vi "Import Invoice data.vi"(0 "Refnum in":T2, 1 "iqa":string, 2 "item_data":T3, 3 "item_data_name":string[](array[string]), 4 "Invoive date":string, 5 "Item no":string, 6 "File data in":string[][](array[string]), 7 "Import Data":T1, 8 "row data":string[](array[string]), 10 "index":i32, 12 "item":string) -> (14 "Refnum out":T2, 15 "File data out":string[][](array[string]), 19 "error out":errorcluster)   [LabVIEW 2017]
uses:
  Control/item colum type.ctl
  <vilib>/addons/database/Connection.llb/Conn ObjectReference.ctl
  <vilib>/addons/database/Connection.llb/Conn Execute.vi
  <vilib>/addons/database/Recordset.llb/Rec Destroy - Connection.vi
  <vilib>/addons/database/Recordset.llb/Rec Fetch Recordset Data (R).vi
  <vilib>/addons/database/_DB Variant To Data/Database Variant To Data.xnode
  <vilib>/addons/database/NI_Database_API.lvlib
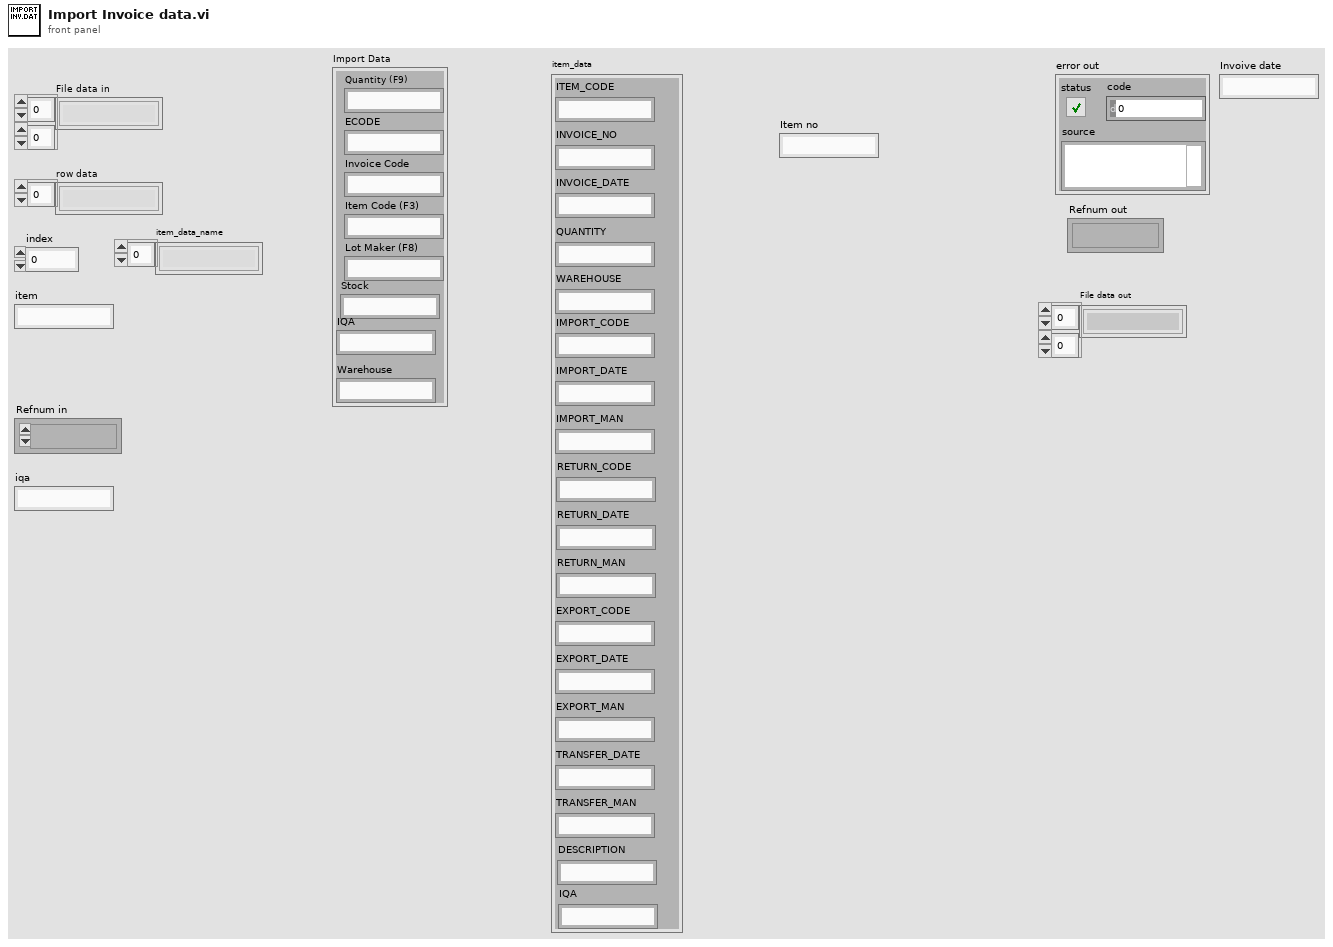
[diagram p1: front panel]
types:
  T1 = cluster{"Quantity (F9)":string, "ECODE":string, "Invoice Code":string, "Item Code (F3)":string, "Lot Maker (F8)":string, "Stock":string, "IQA":string, "Warehouse":string}
  T2 = typedef "NI_Database_API.lvlib/Conn ObjectReference.ctl" = refnum<k1>
  T3 = typedef "item colum type.ctl" = cluster{"ITEM_CODE":string, "INVOICE_NO":string, "INVOICE_DATE":string, "QUANTITY":string, "IMPORT_CODE":string, "IMPORT_DATE":string, "IMPORT_MAN":string, "RETURN_CODE":string, "RETURN_DATE":string, "RETURN_MAN":string, "EXPORT_CODE":string, "EXPORT_DATE":string, "EXPORT_MAN":string, "TRANSFER_DATE":string, "TRANSFER_MAN":string, "DESCRIPTION":string, "IQA":string, "WAREHOUSE":string}
  T4 = cluster{"Item Code (F3)":string, "Invoice Code":string, "Invoive date":string, "Quantity (F9)":string, "Item no":string, "IQA":string, "Lot Maker (F8)":string, "Warehouse":string}
  T5 = typedef "NI_Database_API.lvlib/Rec ObjectReference.ctl" = refnum<k1>
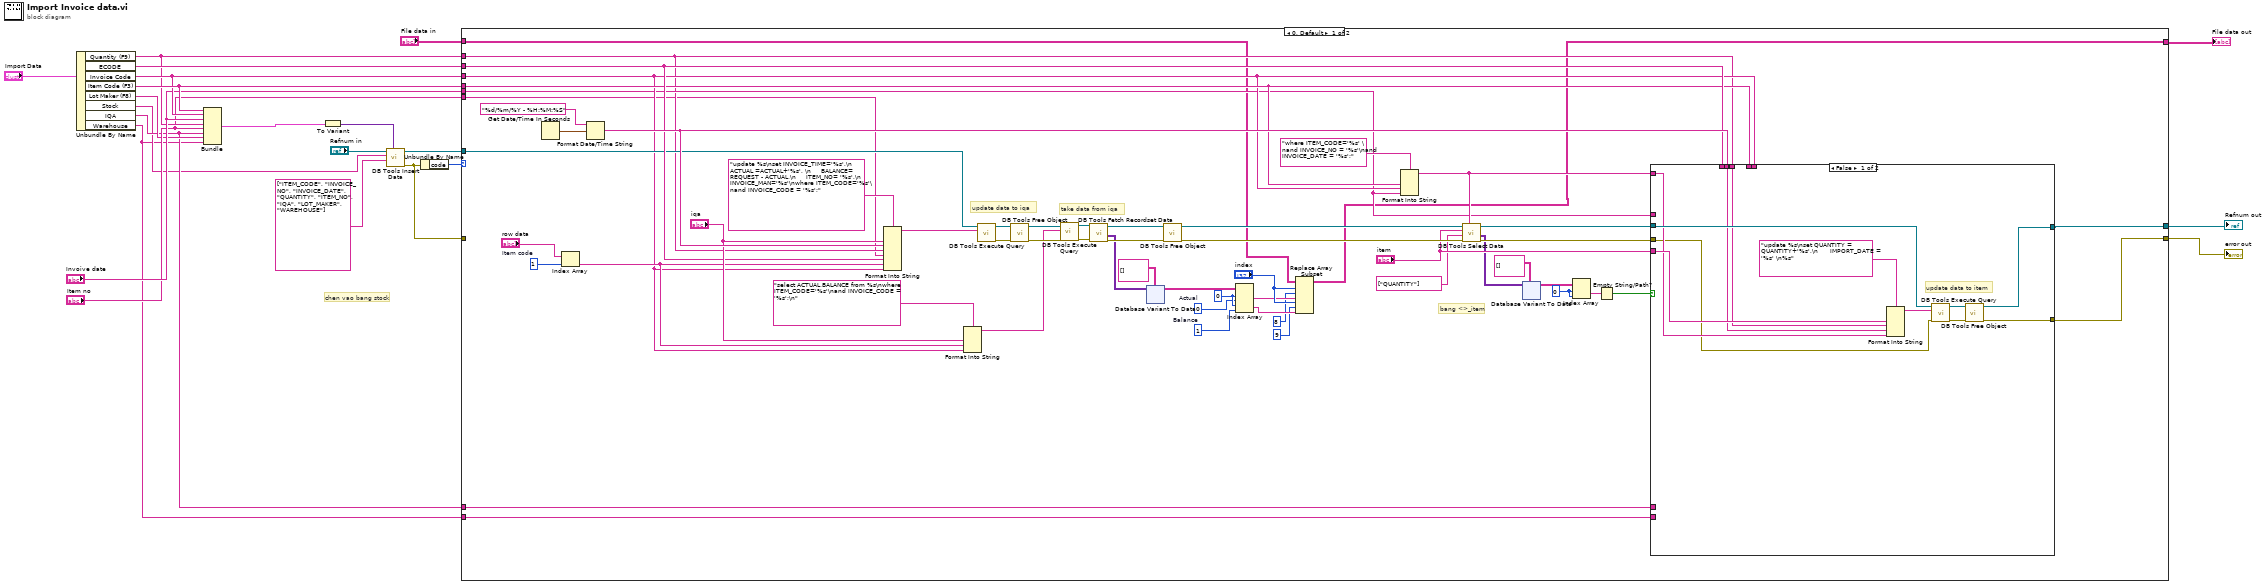
[diagram p0: block diagram]
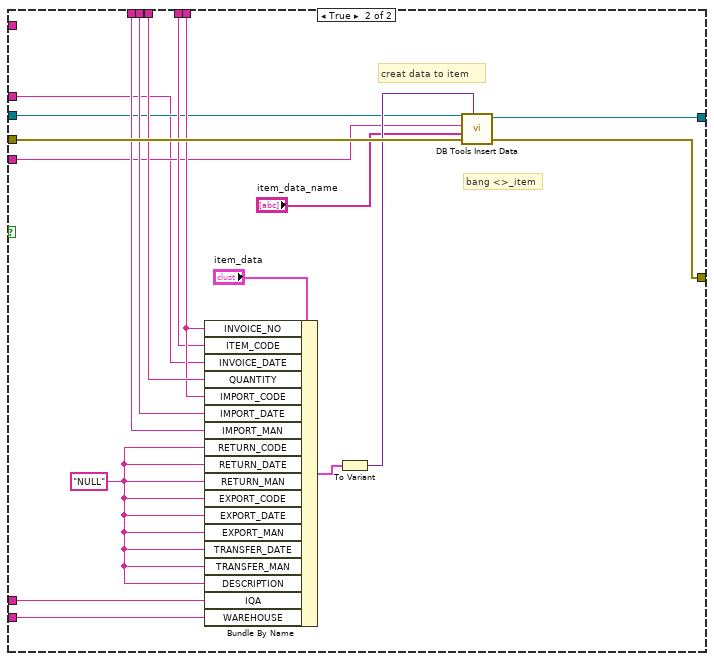
[diagram p2: hidden frame]
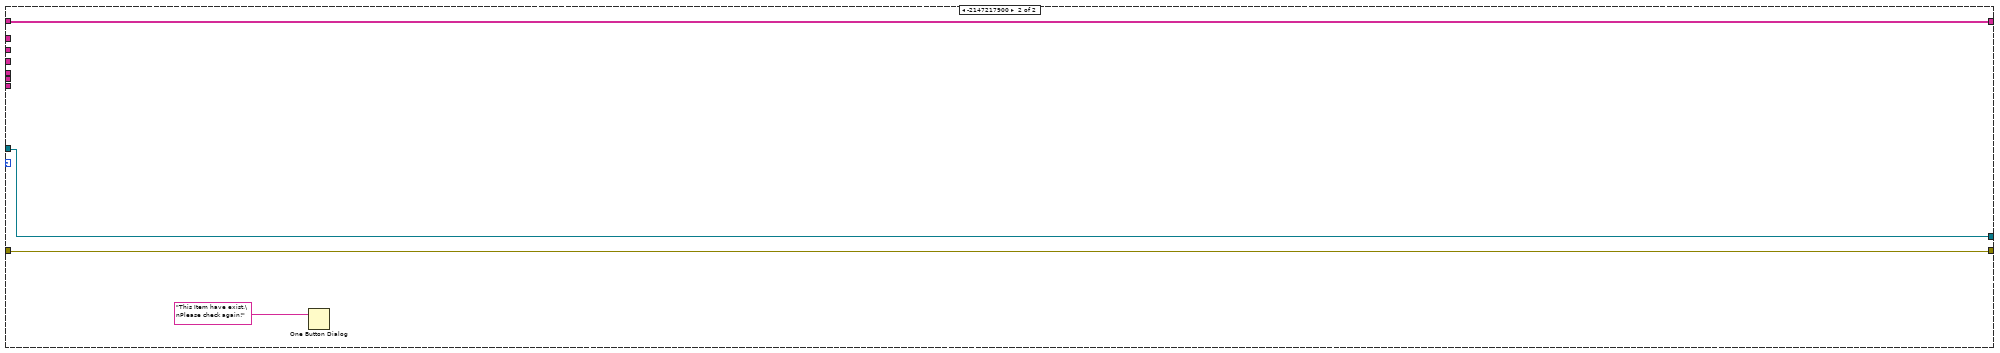
[diagram p3: hidden frame]
diagram:
  # "chen vao bang stock"
  n1 = Unbundle By Name("Import Data") -> ("Quantity (F9)"=w14:string, "ECODE"=w21:string, "Invoice Code"=w16:string, "Item Code (F3)"=w17:string, "Lot Maker (F8)"=w4:string, "Stock"=w2:string, "IQA"=w3:string, "Warehouse"=w1:string)
  n2 = Bundle("Item Code (F3)"=w17, "Invoice Code"=w16, "Invoive date"="Invoive date", "Quantity (F9)"=w14, "Item no"="Item no", "IQA"=w3, "Lot Maker (F8)"=w4, "Warehouse"=w1) -> (w13:T4)  [unwired: 1 in]
  n3 = To Variant(anything=w13) -> (Variant=w12:variant)
  n4 = call <vilib>:"DB Tools Insert Data.vi"("data"=w12, "columns"=string[] ["ITEM_CODE", "INVOICE_NO", "INVOICE_DATE", "QUANTITY", "ITEM_NO", "IQA", "LOT_MAKER", "WAREHOUSE"], "table"=w2, "connection reference"="Refnum in") -> ("error out"=w7:errorcluster, "connection reference out"=w19:T2)  [unwired: 6 in]
  n5 = Unbundle By Name(w7) -> ("code"=w11:i32)
  n6 = case shown="0, Default" w11 {
    tunnel: w21 -> [w46 _]
    tunnel: w19 -> [w34 w198]
    tunnel: w17 -> [w33 _]
    tunnel: w16 -> [w32 _]
    tunnel: "Invoive date" -> [w31 _]
    tunnel: w14 -> [w30 _]
    tunnel: "Item no" -> [w29 _]
    tunnel: w3 -> [w28 _]
    tunnel: "File data in" -> [w27 w199]
    tunnel: [w26 w198] -> w9
    tunnel: [w25 w199] -> w8
    tunnel: w7 -> [_ w197]
    tunnel: [w24 w197] -> w6
    tunnel: w1 -> [w23 _]
    frame 0, Default {
      w39 = 0 ("index (row)")
      w56 = 1  # Balance
      w55 = 0  # Actual
      w78 = 0 ("index (row)")
      w50 = 1  # Item code
      # "bang <>_item"
      # "take data from iqa"
      # "update data to iqa"
      n7 = Get Date/Time In Seconds() -> (seconds since 1Jan1904=w68:timestamp)
      n8 = Index Array(array="row data", index=w50) -> (element=w66:string)
      n9 = Format Date/Time String(time format string (%c)="%d/%m/%Y - %H:%M:%S", seconds (now)=w68) -> (date/time string=w72:string)  [unwired: 1 in]
      n10 = Format Into String(format string="update %s\nset INVOICE_TIME='%s',\n     ACTUAL =ACTUAL+'%s', \n     BALANCE= REQUEST - ACTUAL,\n     ITEM_NO= '%s',\n     INVOICE_MAN='%s'\nwhere ITEM_CODE='%s'\nand INVOICE_CODE = '%s';", "iqa", w72, w30, w29, w46, w66, w32) -> (resulting string=w64:string)  [unwired: 2 in, 1 out]
      n11 = Format Into String(format string="select ACTUAL,BALANCE from %s\nwhere ITEM_CODE='%s'\nand INVOICE_CODE = '%s';\n", "iqa", w66, w32) -> (resulting string=w67:string)  [unwired: 2 in, 1 out]
      n12 = call-poly <vilib>:"DB Tools Execute Query.vi"("SQL query"=w64, "connection reference"=w34) -> ("error out"=w73:errorcluster, "recordset reference"=w62:T5)  [unwired: 6 in]
      n13 = call-poly <vilib>:"DB Tools Free Object.vi"("error in (no error)"=w73, "recordset reference"=w62) -> ("error out"=w74:errorcluster, "connection reference"=w63:T2)  [unwired: 8 in]
      n14 = call-poly <vilib>:"DB Tools Execute Query.vi"("error in (no error)"=w74, "SQL query"=w67, "connection reference"=w63) -> ("error out"=w75:errorcluster, "recordset reference"=w47:T5)  [unwired: 5 in]
      n15 = call-poly <vilib>:"DB Tools Fetch Recordset Data.vi"("error in (no error)"=w75, "recordset reference"=w47) -> ("error out"=w76:errorcluster, "recordset data"=w51:variant[][], "recordset reference out"=w48:T5)  [unwired: 3 in]
      n16 = xnode "Database Variant To Data"("database variant"=w51, "type"=string[][] []) -> ("data"=w53:string[][])  [unwired: 1 in, 1 out]
      n17 = call-poly <vilib>:"DB Tools Free Object.vi"("error in (no error)"=w76, "recordset reference"=w48) -> ("error out"=w77:errorcluster, "connection reference"=w71:T2)  [unwired: 8 in]
      n18 = Index Array(array=w53, index (row) #1=w78, index (col) #1=w55, index (row) #2=w78, index (col) #2=w56) -> (element #1=w59:string, element #2=w60:string)
      n19 = Replace Array Subset "Replace Array Subset"(array=w27, new element #1=w59, index (row) #1="index", index (col) #1=8 ("disabled index (col)"), new element #2=w60, index (row) #2="index", index (col) #2=9 ("disabled index (col)")) -> (w25:string[][])
      n20 = Format Into String(format string="where ITEM_CODE='%s' \nand INVOICE_NO = '%s'\nand INVOICE_DATE = '%s';" ("condition"), w33, w32, w31) -> (resulting string=w35:string)  [unwired: 2 in, 1 out]
      n21 = call <vilib>:"DB Tools Select Data.vi"("condition"=w35, "columns"=string[] ["QUANTITY"], "table"="item", "connection reference"=w71) -> ("data"=w41:variant[][], "connection reference out"=w45:T2)  [unwired: 2 in, 1 out]
      n22 = xnode "Database Variant To Data"("database variant"=w41, "type"=string[][] []) -> ("data"=w40:string[][])  [unwired: 1 in, 1 out]
      n23 = Index Array(array=w40, index (row)=w39, index (col)=w39) -> (element=w38:string)
      n24 = Empty String/Path?(string/path=w38) -> (empty?=w37:bool)
      n25 = case shown="False" w37 {
        tunnel: w77 -> [w80 w108]
        tunnel: w72 -> [w81 w107]
        tunnel: w30 -> [w83 w101]
        tunnel: w46 -> [_ w100]
        tunnel: w32 -> [_ w99]
        tunnel: w33 -> [_ w98]
        tunnel: w45 -> [w86 w97]
        tunnel: "item" -> [w84 w96]
        tunnel: w31 -> [_ w95]
        tunnel: [w85 w94] -> w26
        tunnel: w28 -> [_ w93]
        tunnel: w35 -> [w82 _]
        tunnel: [w79 w92] -> w24
        tunnel: w23 -> [_ w91]
        frame False {
          # "update data to item"
          n26 = Format Into String(format string="update %s\nset QUANTITY = QUANTITY+'%s',\n      IMPORT_DATE = '%s' \n%s", w84, w83, w81, w82) -> (resulting string=w89:string)  [unwired: 2 in, 1 out]
          n27 = call-poly <vilib>:"DB Tools Execute Query.vi"("error in (no error)"=w80, "SQL query"=w89, "connection reference"=w86) -> ("error out"=w90:errorcluster, "recordset reference"=w88:T5)  [unwired: 5 in]
          n28 = call-poly <vilib>:"DB Tools Free Object.vi"("error in (no error)"=w90, "recordset reference"=w88) -> ("error out"=w79:errorcluster, "connection reference"=w85:T2)  [unwired: 8 in]
        }
        frame True {
          w103 = "NULL" ("RETURN_CODE")
          # "bang <>_item"
          # "creat data to item"
          n29 = Bundle By Name(cluster="item_data", "INVOICE_NO"=w99, "ITEM_CODE"=w98, "INVOICE_DATE"=w95, "QUANTITY"=w101, "IMPORT_CODE"=w99, "IMPORT_DATE"=w107, "IMPORT_MAN"=w100, "RETURN_CODE"=w103, "RETURN_DATE"=w103, "RETURN_MAN"=w103, "EXPORT_CODE"=w103, "EXPORT_DATE"=w103, "EXPORT_MAN"=w103, "TRANSFER_DATE"=w103, "TRANSFER_MAN"=w103, "DESCRIPTION"=w103, "IQA"=w93, "WAREHOUSE"=w91) -> (w105:T3)
          n30 = To Variant(anything=w105) -> (Variant=w106:variant)
          n31 = call <vilib>:"DB Tools Insert Data.vi"("data"=w106, "error in (no error)"=w108, "columns"="item_data_name", "table"=w96, "connection reference"=w97) -> ("error out"=w92:errorcluster, "connection reference out"=w94:T2)  [unwired: 5 in]
        }
      }
    }
    frame -2147217900 {
      n32 = One Button Dialog(message="This Item have exist.\nPlease check again!") -> ()  [unwired: 1 in, 1 out]
    }
  }
  "File data out" <- w8
  "Refnum out" <- w9
  "error out" <- w6
